vi "Set homing DSP402.vi"(2 "Done?":bool, 3 "DSP402 in":refnum<class "DSP402.lvclass">) -> (1 "DSP402 out":refnum<class "DSP402.lvclass">)   [LabVIEW 2024, in "canopen.lvlib" / "DSP402.lvclass"]
uses:
  DSP402.lvclass
  DSP402.lvclass/DSP402.ctl
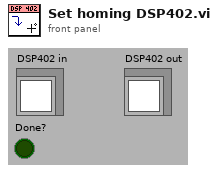
[diagram p1: front panel]
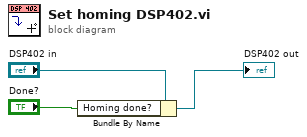
[diagram p0: block diagram]
diagram:
  n1 = Bundle By Name(cluster="DSP402 in", "Homing done?"="Done?") -> (→"DSP402 out":refnum<class "DSP402.lvclass">)
